vi "PXIe-4071_Initialize.vi"(0 "Instrument Info":T1, 1 "User Reference":i32, 5 "error in (no error)":errorcluster) -> (19 "error out":errorcluster)   [LabVIEW 2018, in "PXIe-4071.lvclass"]
uses:
  PXIe-4071.lvclass
  Station/Station Support/Controls/Instrument Info.ctl
  C:/Users/John Gmitter/OneDrive - National Instruments/Git Repo/Harris-FL/Reference Management Server/Instrument Drivers/DMM/DMM Virtual/DMM Virtual.lvclass
  PXIe-4071.lvclass/PXIe-4071.ctl
  DMM Virtual/DMM Virtual.lvclass
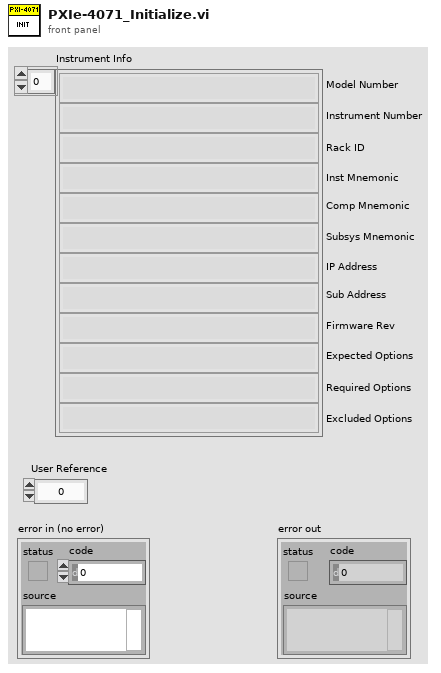
[diagram p1: front panel]
types:
  T1 = typedef "Instrument Info.ctl" = string[]
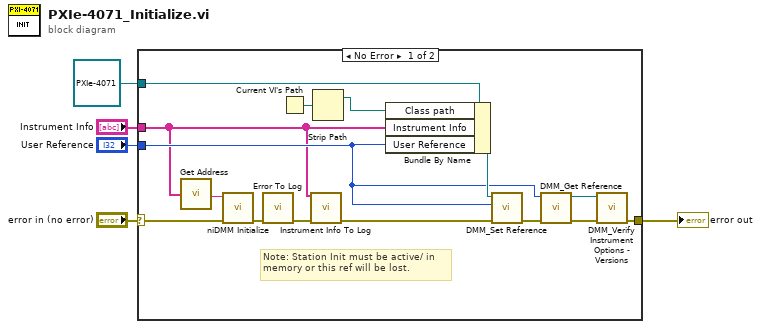
[diagram p0: block diagram]
diagram:
  n1 = case shown="No Error" "error in (no error)" {
    selector: "error in (no error)" -> [w9 w21]
    tunnel: [w16 w21] -> w3
    tunnel: refnum<class "PXIe-4071.lvclass"> refnum ("PXIe-4071.lvclass") -> [w20 _]
    tunnel: "Instrument Info" -> [w11 _]
    tunnel: "User Reference" -> [w14 _]
    frame No Error {
      # "Note: Station Init must be active/ in\nmemory or this ref will be lost."
      n2 = call "Get Address.vi"("Instrument Info"=w11) -> ("Address"=w8:string)  [unwired: 4 in]
      n3 = call <instrlib>:"niDMM Initialize.vi"("error in (no error)"=w9, "Instrument Descriptor"=w8) -> ("error out"=w10:errorcluster)  [unwired: 8 in, 1 out]
      n4 = call "Error To Log.vi"("error in (no error)"=w10) -> ("error out"=w13:errorcluster)  [unwired: 14 in]
      n5 = Current VI's Path() -> (path=w7:path)
      n6 = call "Instrument Info To Log.vi"("Instrument Info"=w11, "error in (no error)"=w13) -> ("error out"=w12:errorcluster)  [unwired: 13 in]
      n7 = Strip Path(path=w7) -> (stripped path=w6:path)  [unwired: 1 out]
      n8 = Bundle By Name(cluster=w20, "Class path"=w6, "Instrument Info"=w11, "User Reference"=w14) -> (w19:refnum<class "PXIe-4071.lvclass">)
      n9 = call "DMM_Set Reference.vi"("error in (no error)"=w12, "Instrument Reference"=w14, "DMM Virtual in"=w19) -> ("error out"=w18:errorcluster)  [unwired: 8 in]
      n10 = call "DMM_Get Reference.vi"("error in (no error)"=w18, "Instrument Reference"=w14) -> ("error out"=w17:errorcluster, "DMM Virtual.lvclass"=w15:refnum<class "DMM Virtual.lvclass">)  [unwired: 7 in, 1 out]
      n11 = call-dynamic "DMM_Verify Instrument Options - Versions.vi"("error in (no error)"=w17, "DMM Virtual in"=w15) -> ("error out"=w16:errorcluster)  [unwired: 8 in, 1 out]
    }
    frame Error {
    }
  }
  "error out" <- w3
